vi "Init ATR Pannel from Excel (SubVI).vi"(10 "name or relative path":string, 11 "Table in":refnum<vi>) -> (2 "TestArray":string[](array[string]))   [LabVIEW 2017]
uses:
  <vilib>/addons/_office/excel.llb/Excel Get Data ([str]).vi
  <vilib>/Utility/NIReport.llb/NI_report.lvclass
  <vilib>/Utility/NIReport.llb/Excel/NI_Excel.lvclass
  <vilib>/addons/_office/NI_ReportGenerationToolkit.lvlib
panel:
  out "size(s)":i32[](array[numeric])
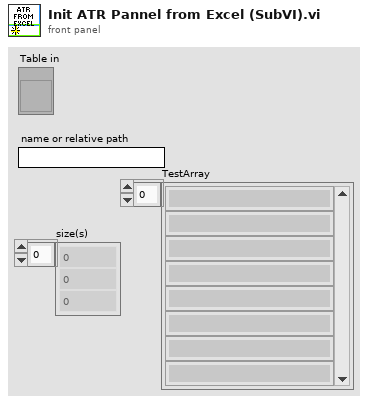
[diagram p1: front panel]
types:
  T1 = enum16{"maximized", "minimized", "normal", "no change"}
  T2 = enum16{"Standard Report", "HTML", "Word", "Excel"}
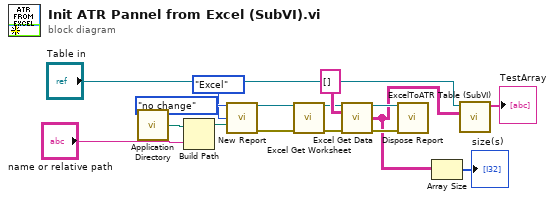
[diagram p0: block diagram]
diagram:
  n1 = call <vilib>:"Application Directory.vi"() -> ("Application Directory"=w12:path)
  n2 = Build Path(base path=w12, name or relative path="name or relative path") -> (appended path=w14:path)
  n3 = call <vilib>:"New Report.vi"("window state (normal)"=T1."no change", "report type"=T2."Excel", "template (empty)"=w14) -> ("report out"=w6:refnum<class "NI_report.lvclass">, "error out"=w5:errorcluster)  [unwired: 11 in]
  n4 = call <vilib>:"Excel Get Worksheet.vi"("report in"=w6, "error in (no error)"=w5) -> ("report out"=w8:refnum<class "NI_report.lvclass">, "error out"=w7:errorcluster)  [unwired: 12 in]
  n5 = call-poly <vilib>:"Excel Get Data.vi"("report in"=w8, "data type"=string[][] [], "error in (no error)"=w7) -> ("report out"=w15:refnum<class "NI_report.lvclass">, "data"=w2:string[][], "error out"=w16:errorcluster)  [unwired: 10 in]
  n6 = call-dynamic "Dispose Report.vi"("report in"=w15, "error in (no error)"=w16) -> ()  [unwired: 13 in, 1 out]
  n7 = Array Size(array=w2) -> (size(s)=→"size(s)":i32[])
  n8 = call "ExcelToATR Table (SubVI).vi"("Shared_strings"=w2, "Table in"="Table in") -> ("TestArray"=→"TestArray":string[])  [unwired: 8 in, 1 out]
